vi "RSZVB Set Advanced Power Transfer Model Frequency State.vi"(8 "error in (no error)":errorcluster {"code" format="%.0x"}, 9 "State (Off)":bool, 10 "Channel (1)":i32=1, 11 "VISA session":refnum<visa-resource-name>) -> (0 "error out":errorcluster {"code" format="%.0x"}, 3 "dup VISA session":refnum<visa-resource-name>)   [LabVIEW 2011]
doc: "This VI enables or disables the advanced power transfer model for frequency converters.\n\nNote(s):This VI overwrites the port specific power transfer model selection; see SOURce<Ch>:POWer<Pt>:CONVerter:TRANsfer:AMODel.\n\nRemote-control command(s):\n[SENSe<Ch>:]CONVerter:AMODel <Boolean>"
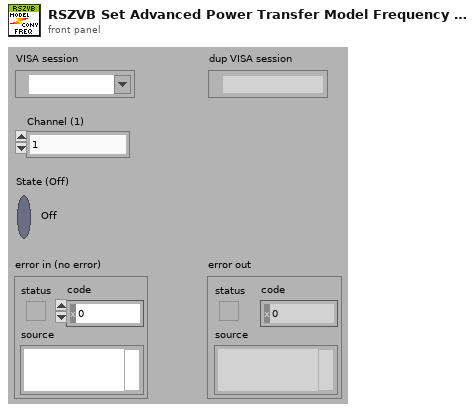
[diagram p1: front panel]
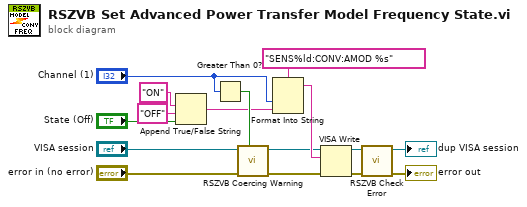
[diagram p0: block diagram]
diagram:
  n1 = Append True/False String(1:"State (Off)", 2:"OFF" ("false string"), 3:"ON" ("true string")) -> (0:w2:string)  [unwired: 1 in]
  n2 = Greater Than 0?(x="Channel (1)") -> (x > 0?=w7:bool)
  n3 = call "RSZVB Coercing Warning.vi"("In Range?"=w7, "error in (no error)"="error in (no error)", "VISA session"="VISA session") -> ("error out"=w13:errorcluster, "dup VISA session"=w12:refnum<visa-resource-name>)  [unwired: 7 in]
  n4 = Format Into String(format string="SENS%ld:CONV:AMOD %s", "Channel (1)", w2) -> (resulting string=w16:string)  [unwired: 2 in, 1 out]
  n5 = VISA Write(VISA resource name=w12, write buffer=w16, error in (no error)=w13) -> (VISA resource name out=w15:refnum<visa-resource-name>, error out=w14:errorcluster)  [unwired: 1 out]
  n6 = call "RSZVB Check Error.vi"("error in (no error)"=w14, "VISA session"=w15) -> ("error out"=→"error out":errorcluster, "dup VISA session"=→"dup VISA session":refnum<visa-resource-name>)  [unwired: 8 in]
